vi "Measure_Voltage.vi"(6 "Resolution in Digits":T1(ring), 8 "error in (no error)":errorcluster, 9 "Range":dbl=1.2, 10 "Level":dbl=1.2, 11 "Measure_Voltage in":refnum<class "Measure_Voltage.lvclass">) -> (0 "error out":errorcluster, 1 "Out of Range":bool, 2 "DC_Voltage":dbl, 3 "Measure_Voltage out":refnum<class "Measure_Voltage.lvclass">)   [LabVIEW 2021, in "Measure_Voltage.lvclass"]
uses:
  Measure_Voltage.lvclass
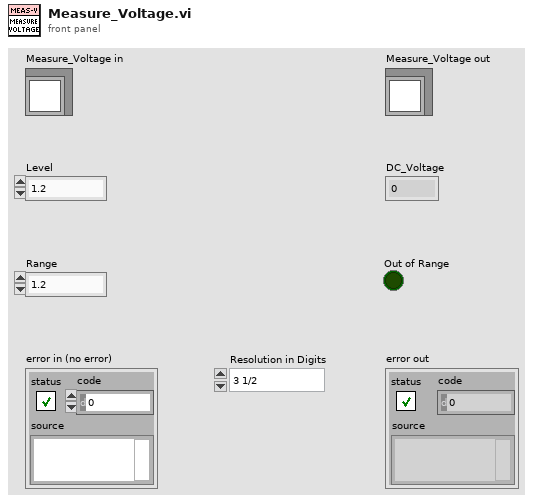
[diagram p1: front panel]
types:
  T1 = enum32{"3 1/2", "4 1/2", "5 1/2", "6 1/2", "7 1/2"}
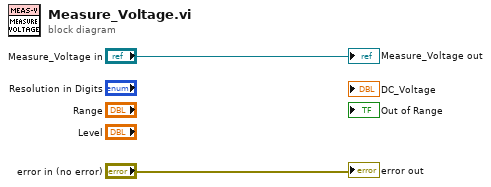
[diagram p0: block diagram]
diagram:
  "error out" <- "error in (no error)"
  "Measure_Voltage out" <- "Measure_Voltage in"
